vi "RichToFlatni_measurementlink_discovery_v1_ServiceLocation.vi"(5 "OutputClusterType":T1, 11 "InputCluster":T2) -> (3 "OutputCluster":T1)   [LabVIEW 2020, in "MeasurementLink Discovery Client.lvlib"]
uses:
  MeasurementLink Discovery Client.lvlib
  ni_measurementlink_discovery_v1_ServiceLocation.ctl
  ni_measurementlink_discovery_v1_ServiceLocation_Flat.ctl
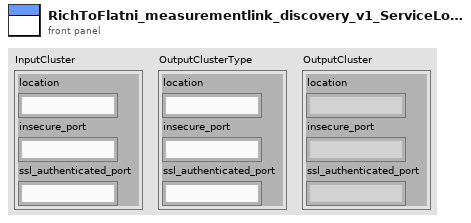
[diagram p1: front panel]
types:
  T1 = typedef "MeasurementLink Discovery Client.lvlib/ni_measurementlink_discovery_v1_ServiceLocation_Flat.ctl" = cluster{"location":string, "insecure_port":string, "ssl_authenticated_port":string}
  T2 = typedef "MeasurementLink Discovery Client.lvlib/ni_measurementlink_discovery_v1_ServiceLocation.ctl" = cluster{"location":string, "insecure_port":string, "ssl_authenticated_port":string}
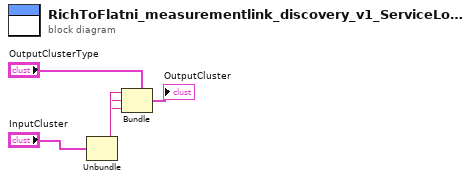
[diagram p0: block diagram]
diagram:
  n1 = Unbundle "Unbundle"("InputCluster") -> ("location"=w3:string, "insecure_port"=w2:string, "ssl_authenticated_port"=w1:string)
  n2 = Bundle "Bundle"(cluster="OutputClusterType", "location"=w3, "insecure_port"=w2, "ssl_authenticated_port"=w1) -> (→"OutputCluster":T1)
